vi "未命名 4.vi"() -> ()   [LabVIEW 2011]
uses:
  Database Connection.lvclass
  Command/Database Command.lvclass
  <vilib>/addons/database/Connection.llb/Conn Set Properties.vi
  <vilib>/addons/database/Auxilliary.llb/DB Tools Format Datetime String (Time Stamp).vi
  <vilib>/addons/database/Recordset.llb/Rec Fetch String Data (R).vi
  <vilib>/addons/database/Command.llb/Cmd Get String Parameter Value (C).vi
  <vilib>/addons/database/Connection.llb/Conn Properties.ctl
panel:
  in  "connection properties":T1
  out "error out":errorcluster caption="错误输出"
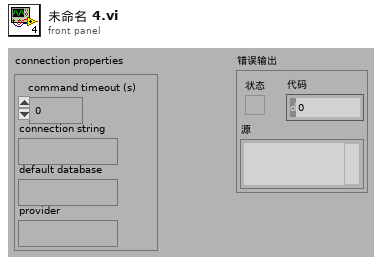
[diagram p1: front panel]
types:
  T1 = typedef "NI_Database_API.lvlib/Conn Properties.ctl" = cluster{"command timeout (s)":i32, "connection string":string, "default database":string, "provider":string}
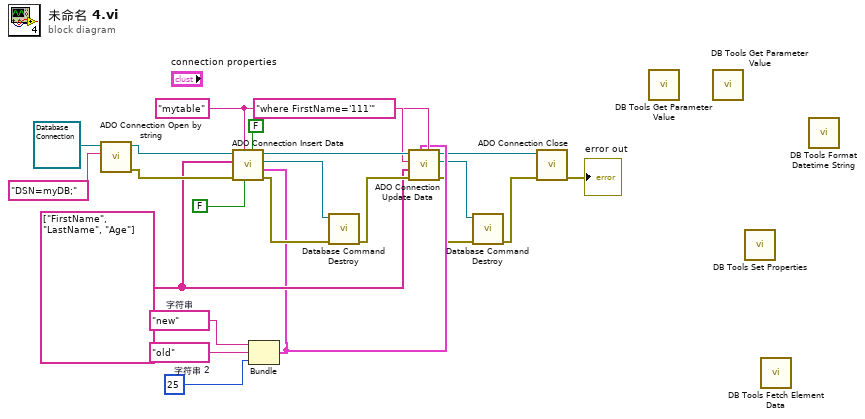
[diagram p0: block diagram]
diagram:
  w13 = "old"  # 字符串 2
  w14 = "new"  # 字符串
  w7 = string[] ["FirstName", "LastName", "Age"] ("columns")
  w8 = "mytable" ("table")
  n1 = call "ADO Connection Open by string.vi"("ConnectionString"="DSN=myDB;", "Database Connection 输入"=refnum<class "Database Connection.lvclass"> refnum ("Database Connection.lvclass")) -> ("error out"=w19:errorcluster, "Database Connection 输出"=w20:refnum<class "Database Connection.lvclass">)  [unwired: 8 in]
  n2 = Bundle("字符串"=w14, "字符串 2"=w13, "数值"=25) -> (w5:cluster{"字符串":string, "字符串 2":string, "数值":i32})  [unwired: 1 in]
  n3 = call "ADO Connection Insert Data.vi"("create table? (F)"=FALSE, "flatten cluster? (F)"=FALSE, "table"=w8, "error in (no error)"=w19, "data"=w5, "columns"=w7, "Database Connection 输入"=w20) -> ("error out"=w17:errorcluster, "Database Command 输出"=w11:refnum<class "Database Command.lvclass">, "Database Connection 输出"=w10:refnum<class "Database Connection.lvclass">)  [unwired: 2 in]
  n4 = call "Database Command Destroy.vi"("error in (no error)"=w17, "Database Command 输入"=w11) -> ("error out"=w9:errorcluster)  [unwired: 8 in, 1 out]
  n5 = call "ADO Connection Update Data.vi"("condition"="where FirstName='111'", "data"=w5, "error in (no error)"=w9, "columns"=w7, "table"=w8, "Database Connection 输入"=w10) -> ("error out"=w4:errorcluster, "Database Command 输出"=w3:refnum<class "Database Command.lvclass">, "Database Connection 输出"=w2:refnum<class "Database Connection.lvclass">)  [unwired: 3 in]
  n6 = call "Database Command Destroy.vi"("error in (no error)"=w4, "Database Command 输入"=w3) -> ("error out"=w1:errorcluster)  [unwired: 8 in, 1 out]
  n7 = call "ADO Connection Close.vi"("error in (no error)"=w1, "Database Connection 输入"=w2) -> ("error out"=→"error out":errorcluster)  [unwired: 9 in]
  n8 = call-poly <vilib>:"DB Tools Get Parameter Value.vi"() -> ()  [unwired: 7 in, 3 out]
  n9 = call-poly <vilib>:"DB Tools Get Parameter Value.vi"() -> ()  [unwired: 7 in, 3 out]
  n10 = call-poly <vilib>:"DB Tools Set Properties.vi"() -> ()  [unwired: 6 in, 2 out]
  n11 = call-poly <vilib>:"DB Tools Fetch Element Data.vi"() -> ()  [unwired: 7 in, 3 out]
  n12 = call-poly <vilib>:"DB Tools Format Datetime String.vi"() -> ()  [unwired: 1 in, 1 out]
